vi "Stop Turnos.vi"(8 "error in (no error)":errorcluster, 11 "User Interface in":refnum<class "User Interface.lvclass">) -> (0 "error out":errorcluster, 3 "User Interface out":refnum<class "User Interface.lvclass">)   [LabVIEW 2020, in "User Interface.lvlib" / "User Interface.lvclass"]
uses:
  User Interface.lvclass
  User Interface.lvclass/User Interface.ctl
  Manejo Turnos Messages/Stop Services Msg/Stop Services Msg.lvclass/Stop Services Msg.ctl
  <vilib>/ActorFramework/Message Enqueuer/Message Enqueuer.lvclass/Message Enqueuer.ctl
  <vilib>/ActorFramework/Message Enqueuer/Enqueue.vi
  Manejo Turnos Messages/Stop Services Msg/Stop Services Msg.lvclass
  C:/Program Files (x86)/National Instruments/LabVIEW 2020/vi.lib/ActorFramework/Message/Message.lvclass
  <vilib>/ActorFramework/Message Priority Queue/Priority Enqueue.vi
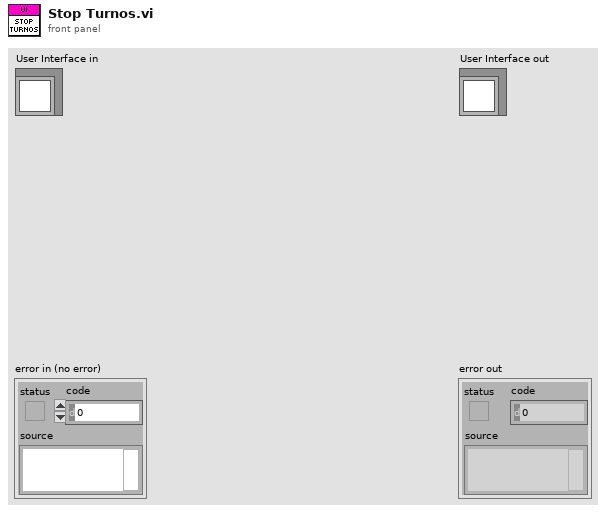
[diagram p1: front panel]
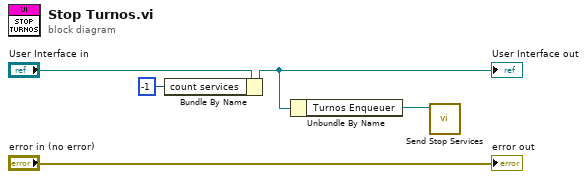
[diagram p0: block diagram]
diagram:
  n1 = Bundle By Name(cluster="User Interface in", "count services"=-1) -> (w2:refnum<class "User Interface.lvclass">)
  "User Interface out" <- w2
  n2 = Unbundle By Name(w2) -> ("Turnos Enqueuer"=w1:refnum<class "Message Enqueuer.lvclass">)
  n3 = call "Send Stop Services.vi"("Message Enqueuer"=w1) -> ()  [unwired: 9 in, 2 out]
  "error out" <- "error in (no error)"
